vi "Do.vi"(8 "error in (no error)":errorcluster, 10 "Actor in":refnum<class "Actor.lvclass">, 11 "Initialize Msg":refnum<class "Initialize Work Msg.lvclass">) -> (0 "error out":errorcluster, 2 "Actor out":refnum<class "Actor.lvclass">)   [LabVIEW 2021, in "Initialize Work Msg.lvclass"]
doc: "This VI delivers the message to the actor by calling the appropriate method(s) on the actor."
uses:
  Initialize Work Msg.lvclass
  <vilib>/ActorFramework/Actor/Actor.lvclass
  Worker/Worker.lvclass
  C:/Program Files/National Instruments/LabVIEW 2021/vi.lib/ActorFramework/Actor/Actor.lvclass
  Initialize Work Msg.lvclass/Initialize Work Msg.ctl
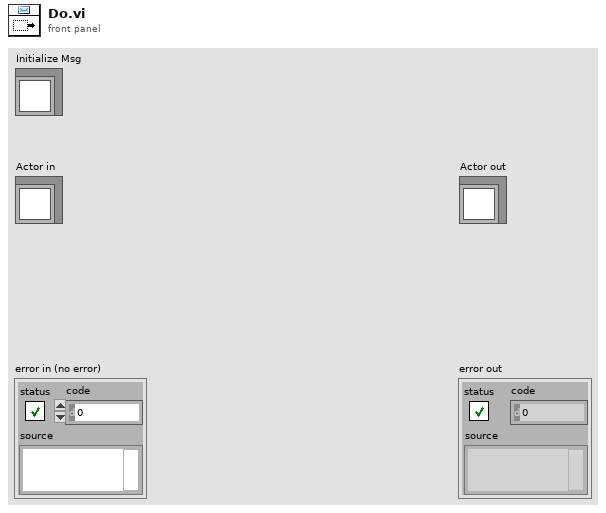
[diagram p1: front panel]
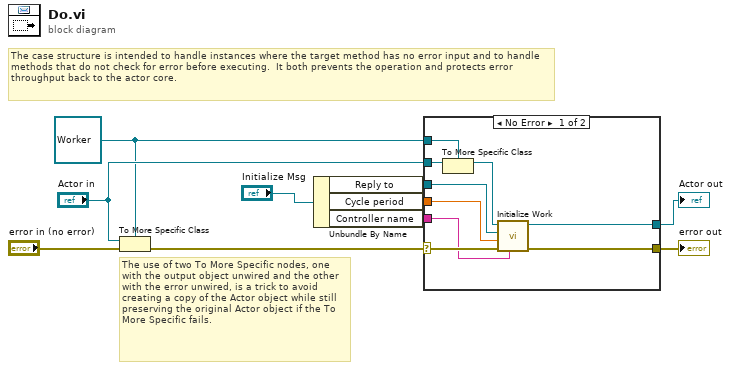
[diagram p0: block diagram]
diagram:
  w5 = refnum<class "Worker.lvclass"> refnum ("Actor in")
  # "The use of two To More Specific nodes, one with the output object unwired and the other with the error unwired, is a trick to avoid creating a copy of the Actor object while still preserving the original Actor object if the To More Specific fails."
  # "The case structure is intended to handle instances where the target method has no error input and to handle methods that do not check for error before executing.  It both prevents the operation and protects error throughput back to the actor core."
  n1 = To More Specific Class(target class=w5, reference="Actor in", error in="error in (no error)") -> (error out=w9:errorcluster)  [unwired: 1 out]
  n2 = Unbundle By Name("Initialize Msg") -> ("Reply to"=w2:refnum<class "Result Reply Msg.lvclass">, "Cycle period"=w3:dbl, "Controller name"=w1:string)
  n3 = case shown="No Error" w9 {
    selector: w9 -> [w17 w21]
    tunnel: [w19 w21] -> w8
    tunnel: [w18 w20] -> w7
    tunnel: "Actor in" -> [w16 w20]
    tunnel: w5 -> [w15 _]
    tunnel: w3 -> [w13 _]
    tunnel: w2 -> [w12 _]
    tunnel: w1 -> [w11 _]
    frame No Error {
      n4 = To More Specific Class(target class=w15, reference=w16) -> (specific class reference=w14:refnum<class "Worker.lvclass">)  [unwired: 1 in, 1 out]
      n5 = call-dynamic "Initialize Work.vi"("Controller name"=w11, "error in (no error)"=w17, "Update period"=w13, "Reply to"=w12, "Measure Object in"=w14) -> ("error out"=w19:errorcluster, "Measure Object out"=w18:refnum<class "Worker.lvclass">)  [unwired: 5 in]
    }
    frame Error {
      # "If type check fails, pass the original object out again."
    }
  }
  "error out" <- w8
  "Actor out" <- w7
